vi "Multiply.vi"(10 "y":dbl, 11 "x":dbl) -> (2 "x*y":dbl)   [LabVIEW 2021]
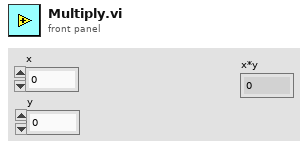
[diagram p1: front panel]
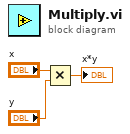
[diagram p0: block diagram]
diagram:
  n1 = Multiply(x="x", y="y") -> (x*y=→"x*y":dbl)
